vi "EMS.vi"() -> (0 "A/DIO4 (Pin 19)":bool)   [LabVIEW 2019]
uses:
  FPGA_subVIs/low level/DIO/DIO enum.ctl
  FPGA_subVIs/low level/DIO/DIO.lvclass
panel:
  out "error out":errorcluster
  in  "error in (no error)":errorcluster
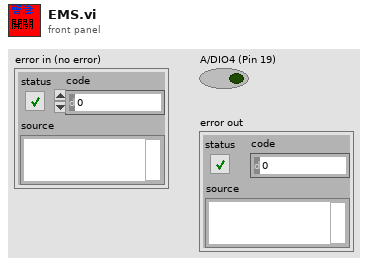
[diagram p1: front panel]
types:
  T1 = typedef "my FPGA lib.lvlib/DIO.lvclass/DIO enum.ctl" = enum16{"US.1", "US.2", "US.3", "US.4", "H.1", "H.2", "H.3", "H.4", "H.5"}
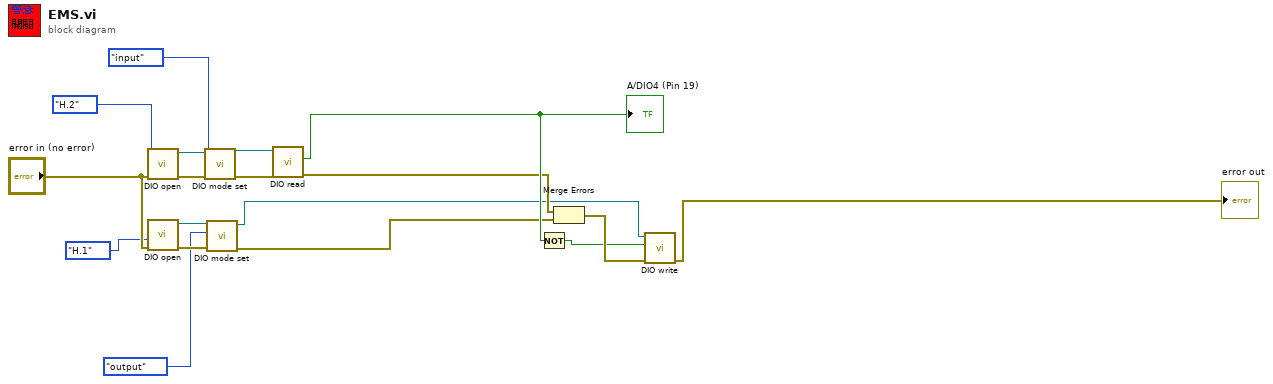
[diagram p0: block diagram]
diagram:
  n1 = call "DIO open.vi"("error in"="error in (no error)", "DIO reference"=DIO_enum."H.2") -> ("error out"=w17:errorcluster, "my FPGA lib.lvlib:DIO.lvclass"=w16:refnum<class "DIO.lvclass">)  [unwired: 8 in]
  n2 = call "DIO open.vi"("error in"="error in (no error)", "DIO reference"=DIO_enum."H.1") -> ("error out"=w11:errorcluster, "my FPGA lib.lvlib:DIO.lvclass"=w10:refnum<class "DIO.lvclass">)  [unwired: 8 in]
  n3 = call "DIO mode set.vi"("error in (no error)"=w17, "mode"=enum16{"input", "output"}."input", "DIO in"=w16) -> ("error out"=w13:errorcluster, "DIO out"=w14:refnum<class "DIO.lvclass">)  [unwired: 7 in]
  n4 = call "DIO mode set.vi"("error in (no error)"=w11, "mode"=enum16{"input", "output"}."output", "DIO in"=w10) -> ("error out"=w5:errorcluster, "DIO out"=w2:refnum<class "DIO.lvclass">)  [unwired: 7 in]
  n5 = call-dynamic "DIO read.vi"("error in (no error)"=w13, "DIO in"=w14) -> ("error out"=w6:errorcluster, "read"=w12:bool)  [unwired: 7 in, 1 out]
  "A/DIO4 (Pin 19)" <- w12
  n6 = Not(x=w12) -> (.not. x?=w3:bool)
  n7 = Merge Errors(w6, w5) -> (w4:errorcluster)
  n8 = call-dynamic "DIO write.vi"("error in (no error)"=w4, "output"=w3, "DIO in"=w2) -> ("error out"=→"error out":errorcluster)  [unwired: 7 in, 1 out]
